vi "ConvertTo(error).vi"(8 "error in":errorcluster, 9 "Message Payload":variant) -> (0 "error out":errorcluster, 1 "Message Payload error":errorcluster)   [LabVIEW 2018]
doc: "Convert variant to error cluster\n\nBolder Software LLC"
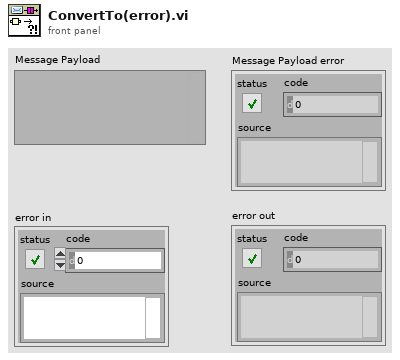
[diagram p1: front panel]
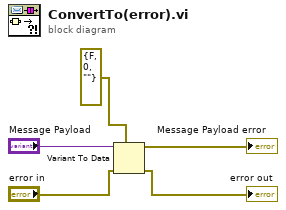
[diagram p0: block diagram]
diagram:
  n1 = Variant To Data(error in="error in", type=errorcluster {"status"=FALSE, "code"=0, "source"=""} ("Message Payload error"), Variant="Message Payload") -> (data=→"Message Payload error":errorcluster, error out=→"error out":errorcluster)
